vi "SendParameter2Variable.vi"(0 "Shared Variable":refnum<k21>, 1 "Parameter":variant, 2 "typeDescriptor":string, 3 "ms timeout (0)":i32, 5 "error in (no error)":errorcluster) -> (17 "timed out":bool, 19 "error out":errorcluster)   [LabVIEW 2012, in "HGF_DSC.lvlib" / "HGF_DSCService.lvclass"]
uses:
  HGF_DSCService.lvclass
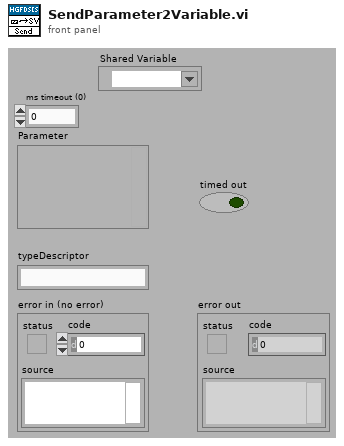
[diagram p1: front panel]
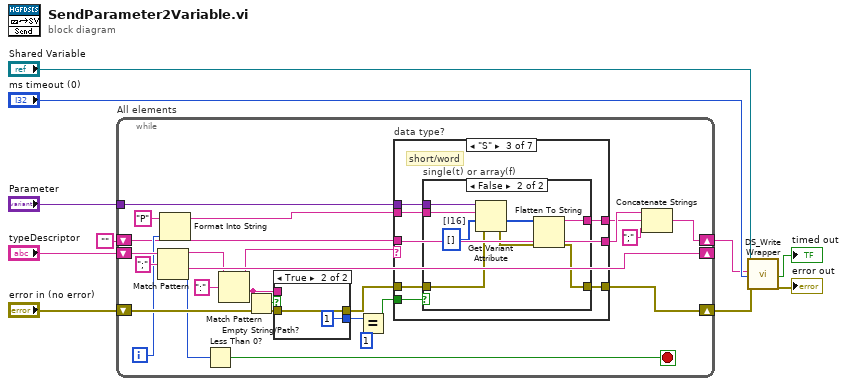
[diagram p0: block diagram]
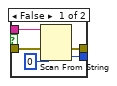
[diagram p2: hidden frame]
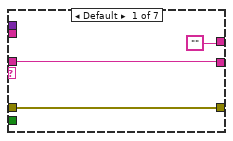
[diagram p3: hidden frame]
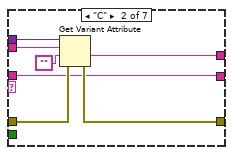
[diagram p4: hidden frame]
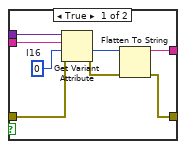
[diagram p5: hidden frame]
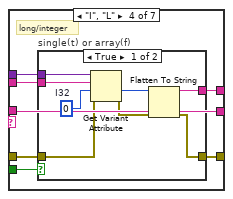
[diagram p6: hidden frame]
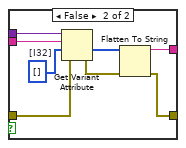
[diagram p7: hidden frame]
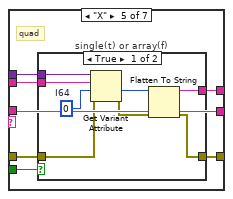
[diagram p8: hidden frame]
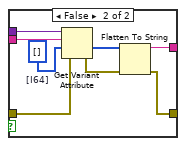
[diagram p9: hidden frame]
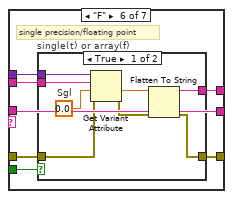
[diagram p10: hidden frame]
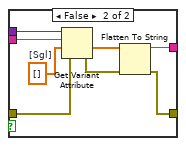
[diagram p11: hidden frame]
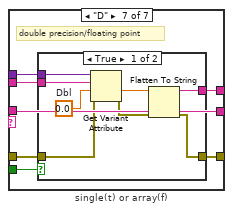
[diagram p12: hidden frame]
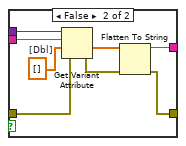
[diagram p13: hidden frame]
diagram:
  n1 = while "All elements" {
    shift-right: [w32] -> _
    shift-left: "typeDescriptor" -> [w34]
    shift-right: [w22] -> w3
    shift-left: "error in (no error)" -> [w35]
    tunnel: "Parameter" -> [w21]
    shift-right: [w16] -> w4
    shift-left: "" -> [w17]
    i -> [w26]
    stop <- w31 stop-if-true
    n2 = Match Pattern(string=w34, regular expression=";") -> (before substring=w29:string, after substring=w32:string, offset past match=w30:i32)  [unwired: 2 out]
    n3 = Format Into String(initial string="P", w26) -> (resulting string=w25:string)  [unwired: 2 in, 1 out]
    n4 = Less Than 0?(x=w30) -> (x < 0?=w31:bool)
    n5 = Match Pattern(string=w29, regular expression=":") -> (before substring=w24:string, after substring=w11:string)  [unwired: 3 out]
    n6 = Empty String/Path?(string/path=w11) -> (empty?=w12:bool)
    n7 = case shown="True" w12 {
      tunnel: w11 -> [w39 _]
      tunnel: w35 -> [w38 w42]
      tunnel: [w37 w42] -> w23
      tunnel: [w36 1 ("default value 1")] -> w20
      frame False {
        n8 = Scan From String(input string=w39, error in=w38, default 1=0 ("default value 1")) -> (error out=w37:errorcluster, output 1=w36:i32)  [unwired: 2 in, 2 out]
      }
      frame True {
      }
    }
    n9 = Equal?(x=w20, y=1) -> (x = y?=w18:bool)
    n10 = case "data type?" shown="\"S\"" w24 {
      tunnel: w25 -> [_ w50 w57 w80 w103 w126 w149]
      tunnel: w23 -> [w45 w51 w58 w81 w104 w127 w150]
      tunnel: [w45 w48 w56 w79 w102 w125 w148] -> w22
      tunnel: w21 -> [_ w52 w59 w82 w105 w128 w151]
      tunnel: w18 -> [_ _ w55 w78 w101 w124 w147]
      tunnel: [w44 w47 w53 w76 w99 w122 w145] -> w15
      tunnel: w17 -> [w44 w47 w53 w76 w99 w122 w145]
      tunnel: ["" w46 w54 w77 w100 w123 w146] -> w14
      frame Default {
      }
      frame "C" {
        n11 = Get Variant Attribute(Variant=w52, name=w50, default value (empty Variant)="", error in=w51) -> (value=w46:string, error out=w48:errorcluster)  [unwired: 2 out]
      }
      frame "S" {
        # "short/word"
        n12 = case "single(t) or array(f)" shown="False" w55 {
          tunnel: w59 -> [w67 w75]
          tunnel: w58 -> [w66 w74]
          tunnel: w57 -> [w65 w73]
          tunnel: [w62 w68] -> w56
          tunnel: [w61 w71] -> w54
          frame True {
            w64 = i16 0  # I16
            n13 = Get Variant Attribute(Variant=w67, name=w65, default value (empty Variant)=w64, error in=w66) -> (value=w60:i16, error out=w63:errorcluster)  [unwired: 2 out]
            n14 = Flatten To String(anything=w60, error in (no error)=w63) -> (data string=w61:string, error out=w62:errorcluster)  [unwired: 3 out]
          }
          frame False {
            w72 = i16[] []  # [I16]
            n15 = Get Variant Attribute(Variant=w75, name=w73, default value (empty Variant)=w72, error in=w74) -> (value=w70:i16[], error out=w69:errorcluster)  [unwired: 2 out]
            n16 = Flatten To String(anything=w70, error in (no error)=w69) -> (data string=w71:string, error out=w68:errorcluster)  [unwired: 3 out]
          }
        }
      }
      frame "I", "L" {
        # "long/integer"
        n17 = case "single(t) or array(f)" shown="True" w78 {
          tunnel: w82 -> [w90 w98]
          tunnel: w81 -> [w89 w97]
          tunnel: w80 -> [w88 w96]
          tunnel: [w85 w91] -> w79
          tunnel: [w84 w94] -> w77
          frame True {
            w87 = 0  # I32
            n18 = Get Variant Attribute(Variant=w90, name=w88, default value (empty Variant)=w87, error in=w89) -> (value=w83:i32, error out=w86:errorcluster)  [unwired: 2 out]
            n19 = Flatten To String(anything=w83, error in (no error)=w86) -> (data string=w84:string, error out=w85:errorcluster)  [unwired: 3 out]
          }
          frame False {
            w95 = i32[] []  # [I32]
            n20 = Get Variant Attribute(Variant=w98, name=w96, default value (empty Variant)=w95, error in=w97) -> (value=w93:i32[], error out=w92:errorcluster)  [unwired: 2 out]
            n21 = Flatten To String(anything=w93, error in (no error)=w92) -> (data string=w94:string, error out=w91:errorcluster)  [unwired: 3 out]
          }
        }
      }
      frame "X" {
        # "quad"
        n22 = case "single(t) or array(f)" shown="True" w101 {
          tunnel: w105 -> [w113 w121]
          tunnel: w104 -> [w112 w120]
          tunnel: w103 -> [w111 w119]
          tunnel: [w108 w114] -> w102
          tunnel: [w107 w117] -> w100
          frame True {
            w110 = i64 0  # I64
            n23 = Get Variant Attribute(Variant=w113, name=w111, default value (empty Variant)=w110, error in=w112) -> (value=w106:i64, error out=w109:errorcluster)  [unwired: 2 out]
            n24 = Flatten To String(anything=w106, error in (no error)=w109) -> (data string=w107:string, error out=w108:errorcluster)  [unwired: 3 out]
          }
          frame False {
            w118 = i64[] []  # [I64]
            n25 = Get Variant Attribute(Variant=w121, name=w119, default value (empty Variant)=w118, error in=w120) -> (value=w116:i64[], error out=w115:errorcluster)  [unwired: 2 out]
            n26 = Flatten To String(anything=w116, error in (no error)=w115) -> (data string=w117:string, error out=w114:errorcluster)  [unwired: 3 out]
          }
        }
      }
      frame "F" {
        # "single precision/floating point"
        n27 = case "single(t) or array(f)" shown="True" w124 {
          tunnel: w128 -> [w136 w144]
          tunnel: w127 -> [w135 w143]
          tunnel: w126 -> [w134 w142]
          tunnel: [w131 w137] -> w125
          tunnel: [w130 w140] -> w123
          frame True {
            w133 = sgl 0.0  # Sgl
            n28 = Get Variant Attribute(Variant=w136, name=w134, default value (empty Variant)=w133, error in=w135) -> (value=w129:sgl, error out=w132:errorcluster)  [unwired: 2 out]
            n29 = Flatten To String(anything=w129, error in (no error)=w132) -> (data string=w130:string, error out=w131:errorcluster)  [unwired: 3 out]
          }
          frame False {
            w141 = sgl[] []  # [Sgl]
            n30 = Get Variant Attribute(Variant=w144, name=w142, default value (empty Variant)=w141, error in=w143) -> (value=w139:sgl[], error out=w138:errorcluster)  [unwired: 2 out]
            n31 = Flatten To String(anything=w139, error in (no error)=w138) -> (data string=w140:string, error out=w137:errorcluster)  [unwired: 3 out]
          }
        }
      }
      frame "D" {
        # "double precision/floating point"
        n32 = case "single(t) or array(f)" shown="True" w147 {
          tunnel: w151 -> [w159 w167]
          tunnel: w150 -> [w158 w166]
          tunnel: w149 -> [w157 w165]
          tunnel: [w154 w160] -> w148
          tunnel: [w153 w163] -> w146
          frame True {
            w156 = 0.0  # Dbl
            n33 = Get Variant Attribute(Variant=w159, name=w157, default value (empty Variant)=w156, error in=w158) -> (value=w152:dbl, error out=w155:errorcluster)  [unwired: 2 out]
            n34 = Flatten To String(anything=w152, error in (no error)=w155) -> (data string=w153:string, error out=w154:errorcluster)  [unwired: 3 out]
          }
          frame False {
            w164 = dbl[] []  # [Dbl]
            n35 = Get Variant Attribute(Variant=w167, name=w165, default value (empty Variant)=w164, error in=w166) -> (value=w162:dbl[], error out=w161:errorcluster)  [unwired: 2 out]
            n36 = Flatten To String(anything=w162, error in (no error)=w161) -> (data string=w163:string, error out=w160:errorcluster)  [unwired: 3 out]
          }
        }
      }
    }
    n37 = Concatenate Strings(w15, w14, ";" ("string")) -> (w16:string)
  }
  n38 = call "DS_Write Wrapper.vi"("Shared Variable"="Shared Variable", "rawData"=w4, "ms timeout (0)"="ms timeout (0)", "error in"=w3) -> ("timed out"=→"timed out":bool, "error out"=→"error out":errorcluster)  [unwired: 14 out]
